vi "integrator2.vi"(1 "reverse intergral":bool, 2 "set ends to 0?":bool, 3 "renormalization":dbl=1.0, 4 "pretrigger t":dbl=1.0, 5 "dt":dbl=1.0, 6 "data":dbl[](array[numeric])) -> (0 "integrated data":dbl[](array[numeric]))   [LabVIEW 2015]
uses:
  <vilib>/Analysis/baseanly.llb/Mean (DBL).vi
  <vilib>/Analysis/NI_AALBase.lvlib
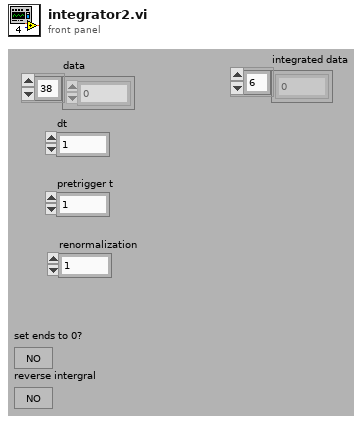
[diagram p1: front panel]
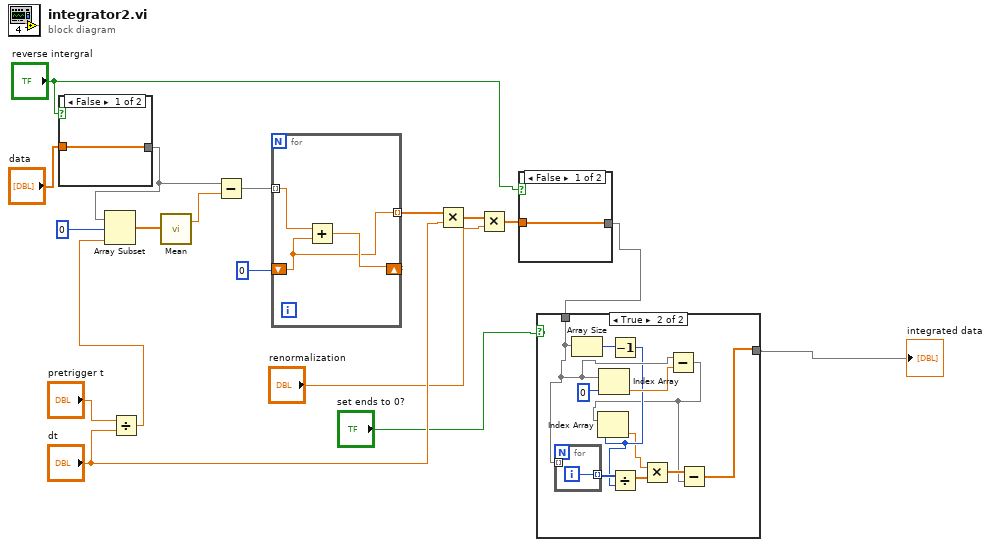
[diagram p0: block diagram]
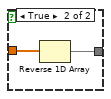
[diagram p3: hidden frame]
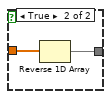
[diagram p4: hidden frame]
diagram:
  n1 = case shown="False" "reverse intergral" {
    tunnel: "data" -> [w19 w21]
    tunnel: [w19 w20] -> w13
    frame False {
    }
    frame True {
      n2 = Reverse 1D Array(array=w21) -> (reversed array=w20:dbl[])
    }
  }
  n3 = Divide(x="pretrigger t", y="dt") -> (x/y=w17:dbl)
  n4 = Array Subset(array=w13, index=0, length=w17) -> (w14:dbl[])
  n5 = call-poly <vilib>:"Mean.vi"("X"=w14) -> ("mean"=w1:dbl)  [unwired: 1 out]
  n6 = Subtract(x=w13, y=w1) -> (x-y=w12:dbl[])
  n7 = for {
    tunnel: w12 -> [w24] mode=indexing
    shift-right: [w23] -> _
    shift-left: 0 -> [w22]
    tunnel: [w22] -> w10 mode=indexing
    n8 = Add(x=w24, y=w22) -> (x+y=w23:dbl)
  }
  n9 = Multiply(x=w10, y="dt") -> (x*y=w8:dbl[])
  n10 = Multiply(x=w8, y="renormalization") -> (x*y=w6:dbl[])
  n11 = case shown="False" "reverse intergral" {
    tunnel: w6 -> [w25 w27]
    tunnel: [w25 w26] -> w3
    frame False {
    }
    frame True {
      n12 = Reverse 1D Array(array=w27) -> (reversed array=w26:dbl[])
    }
  }
  n13 = case shown="True" "set ends to 0?" {
    tunnel: w3 -> [w28 w36]
    tunnel: [w28 w29] -> w2
    frame False {
    }
    frame True {
      n14 = for {
        tunnel: w36 -> [_] mode=indexing
        tunnel: [w40] -> w35 mode=indexing
        i -> [w40]
      }
      n15 = Array Size(array=w36) -> (size(s)=w39:i32)
      n16 = Index Array(array=w36, index=0) -> (element=w37:dbl)
      n17 = Decrement(x=w39) -> (x-1=w34:i32)
      n18 = Divide(x=w35, y=w34) -> (x/y=w33:dbl[])
      n19 = Subtract(x=w36, y=w37) -> (x-y=w30:dbl[])
      n20 = Index Array(array=w30, index=w34) -> (element=w32:dbl)
      n21 = Multiply(x=w32, y=w33) -> (x*y=w31:dbl[])
      n22 = Subtract(x=w31, y=w30) -> (x-y=w29:dbl[])
    }
  }
  "integrated data" <- w2
